vi "CIPT_softwarecontrol 24 7 23.vi"() -> ()   [LabVIEW 2022 SP3]
uses:
  CIPT modes.ctl
  <vilib>/Analysis/baseanly.llb/Mean (DBL).vi
  <vilib>/Utility/file.llb/Read Delimited Spreadsheet (DBL).vi
  <vilib>/Utility/file.llb/Read Delimited Spreadsheet (I64).vi
  <vilib>/gmath/NumericalOptimization/Nonlinear Curve Fit LM.vi
  <vilib>/Utility/file.llb/Write Delimited Spreadsheet (string).vi
  C:/CIPT/Labview Project/Camera Driver/Labview Driver/OtherDrivers/LabVIEW/ueye.NET/uEyeDotNet.dll
  CIPT/Labview Project/Camera Driver/Labview Driver/OtherDrivers/LabVIEW/ueye.NET/uEyeDotNet.dll
  <vilib>/Utility/file.llb/Write Delimited Spreadsheet (DBL).vi
  <vilib>/Utility/file.llb/Write Delimited Spreadsheet (I64).vi
  <vilib>/gmath/NI_Gmath.lvlib
  <instrlib>/Keithley DMM6500 DAQ6500 Series/Keithley DMM6500 DAQ6500 Series.lvlib
  <instrlib>/Keithley 24XX/Keithley 24XX.lvlib
  <instrlib>/Keithley 2182/Keithley 2182.lvlib
  <vilib>/Analysis/NI_AALBase.lvlib
panel:
  out "Comms Errors":errorcluster[](array[cluster])
  in  "Save Filr":bool
  out "error file out":errorcluster
  in  "output file path":path=path "C:/CIPT/Labview Project/csv files/test output.csv"
  in  "stop":bool
  in  "Tab Control":T1(tab)
  in  "Camera ID 3":enum16{"2", "1"}(ring)
  in  "Camera ID 1":enum16{"2", "1"}(ring)
  in  "down a2":bool
  in  "up a2":bool
  in  "down a1":bool
  in  "up a1":bool
  in  "down a3":bool
  in  "up a3":bool
  in  "down all":bool
  in  "up all":bool
  in  "steps /\n continuous \ntoggle":bool
  out "Image first camera":picture
  out "Serial Number 1":string
  in  "Init Camera":bool
  in  "Exit Camera":bool
  in  "Init Camera 2":bool
  in  "Exit Camera 2":bool
  out "Serial Number 2":string
  out "Image second camera":picture
  out "Error Camera 1":errorcluster caption="error"
  out "Error Camera 2":errorcluster caption="error"
  in  "COM 1":refnum<visa-resource-name>
  out "error":errorcluster
  in  "Probe Landing File":path=path "C:/CIPT/Labview Project/csv files/Probe Landing cipt.csv"
  in  "Landing Test on/off?":bool
  in  "load file":bool
  in  "Step size":i32=10
  out "Resistance":dbl[][](array[numeric])
  out "Measurment":sgl[](array[numeric])
  out "Loaded":bool
  out "Loaded":bool
  out "Error Probe Configuration File":errorcluster
  in  "Probe Configuration File":path=path "C:/CIPT/Labview Project/csv files/test probe config.csv"
  in  "Probe Settings File":path=path "C:/CIPT/Labview Project/csv files/deafult_probe_setrings.CSV"
  out "Error Probe Settings File":errorcluster
  out "Probe Spacings":dbl[][](array[numeric])
  in  "Load":bool
  in  "Multiplexer":refnum<visa-resource-name>
  out "all rows":i64[][](array[numeric])
  out "Results Description":string[](array[string])
  out "Results":dbl[][](array[numeric])
  out "Probe Set 2":i32
  in  "Compliance voltage (V)":dbl=42.0
  in  "Measure Instrument":refnum<visa-resource-name>
  in  "Radio Buttons":T2 caption="Select Instrumentation"
  in  "Source Instrument":refnum<visa-resource-name>
  in  "Run":bool
  in  "Current (µA)":dbl=10.0
  out "Measurement Log":string
  out "Probe Set":i32
  in  "Measurement Repeats":i32=10
  in  "Top Film R est.":dbl=0.25
  in  "Bottm Film R est.":dbl=0.25
  in  "RA est.":dbl=0.25
  out "Top Film R":dbl
  out "Bottom Film R":dbl
  out "RA":dbl
  out "error out (fitting model)":errorcluster
  in  "Fit Data":bool
  out "Measurements Map Out":map{string, dbl[]}(c390)
  # "Probe Landing cipt_probe check: checks probes individually \nProbe Landing cipt: checks for any connection"
  # "All"
  # "End"
  # "home"
  # "Delete"
  # "Insert"
  # "Page Down"
  # "Page up"
  # "F2"
  # "F1"
  # "Steps"
  # "Continuous"
  # "Probe Settings"
  # "Probe Configuration"
  # "I+"
  # "V+"
  # "V-"
  # "I-"
  # "Max Resolution of 2400 is 300 µV in 200 mV range"
  # "/"
  # "Sheet Resistance (RA)"
  # "Estimated Values"
  # "Fitted Values"
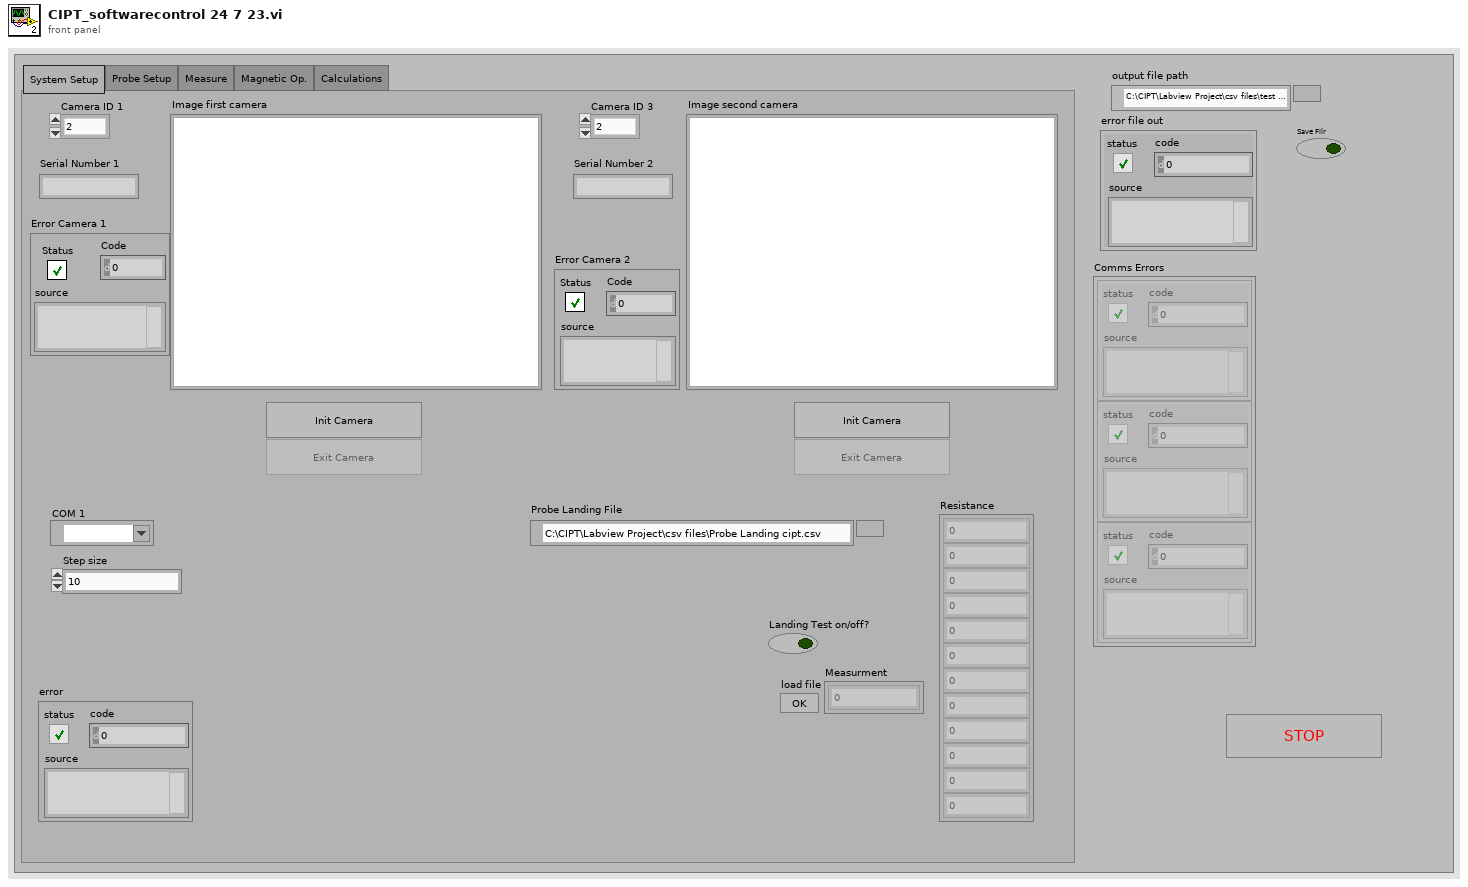
[diagram p1: front panel]
types:
  T1 = enum32{"System Setup", "Probe Setup", "Measure", "Magnetic Op.", "Calculations"}
  T2 = typedef "CIPT modes.ctl" = enum32{"DAQ6510", "2400 Only", "2400 and  2182", "SR830", "SR830 and 6221"}
  T3 = enum32{"System Setup", "Probe Setup", "Measure", "Magnetic Operations", "Calculations + Analyis"}
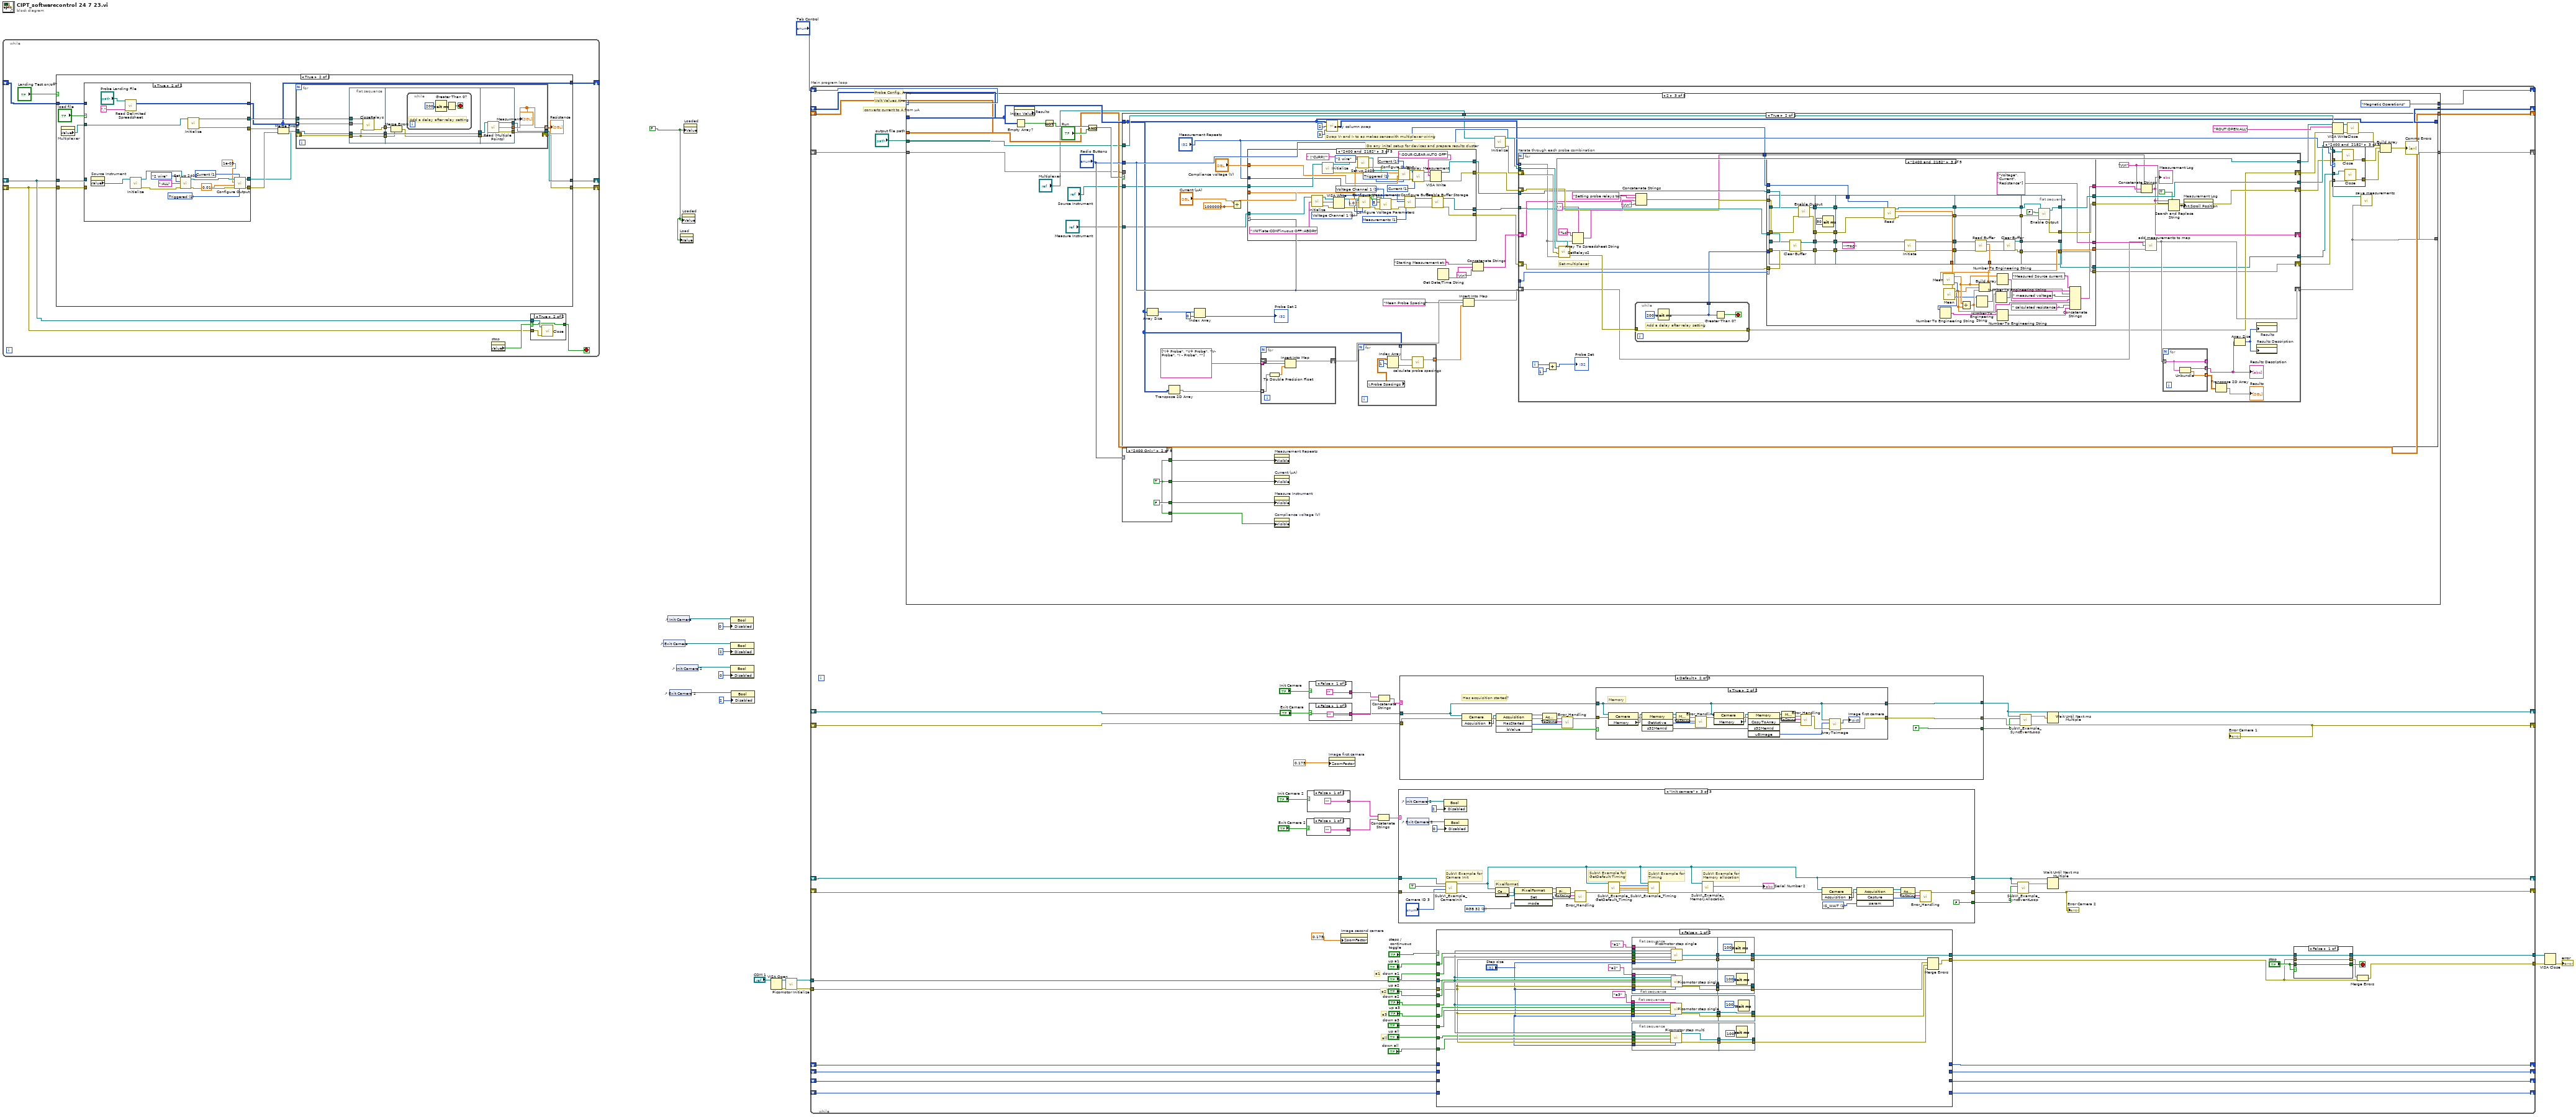
[diagram p0: block diagram]
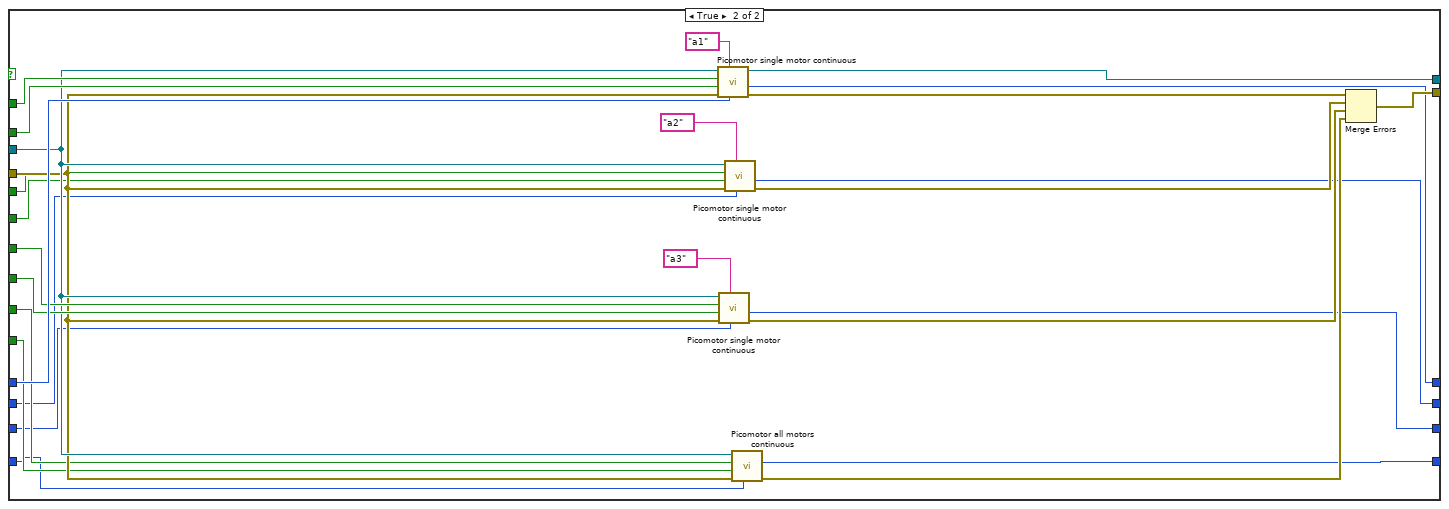
[diagram p5: hidden frame]
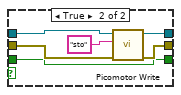
[diagram p6: hidden frame]
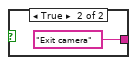
[diagram p7: hidden frame]
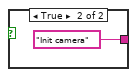
[diagram p8: hidden frame]
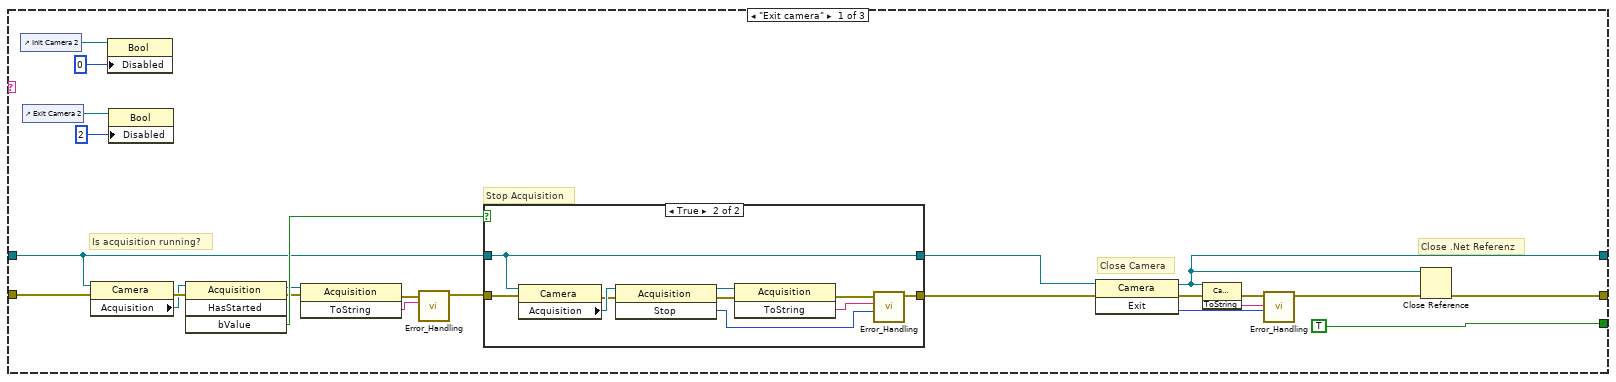
[diagram p9: hidden frame]
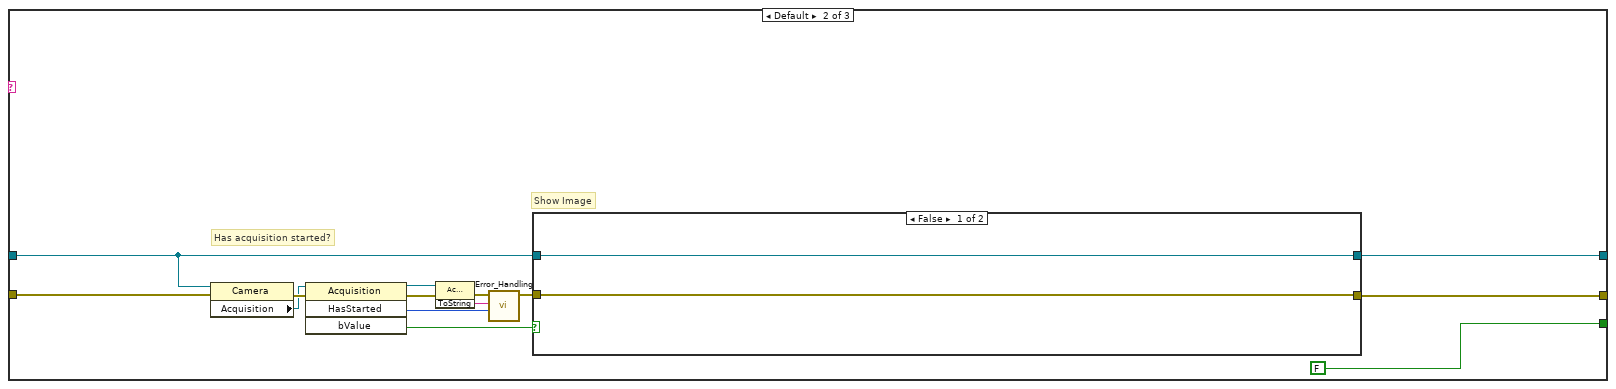
[diagram p11: hidden frame]
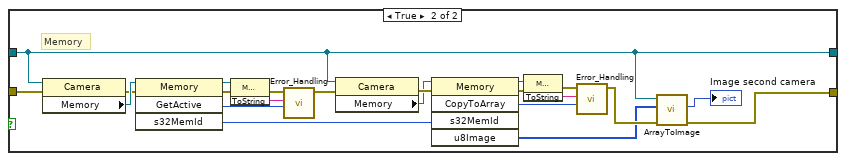
[diagram p12: hidden frame]
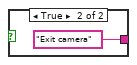
[diagram p13: hidden frame]
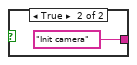
[diagram p14: hidden frame]
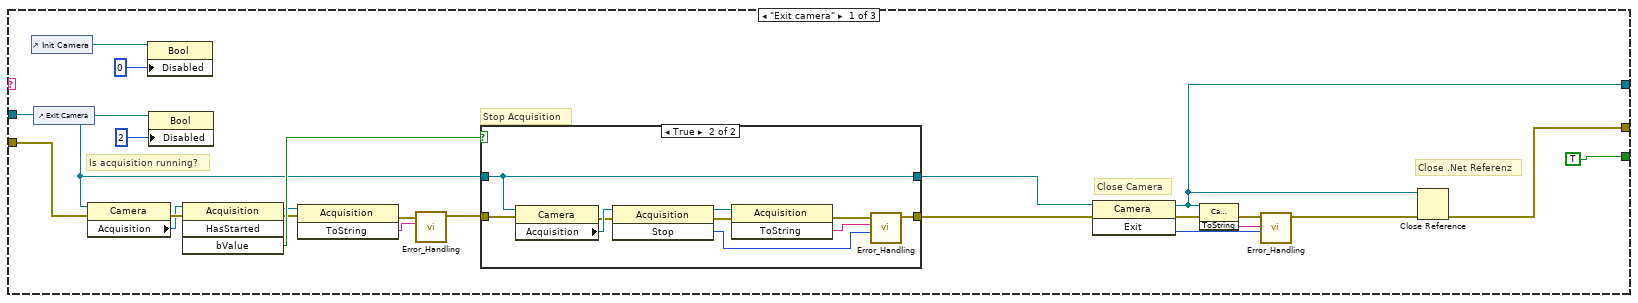
[diagram p15: hidden frame]
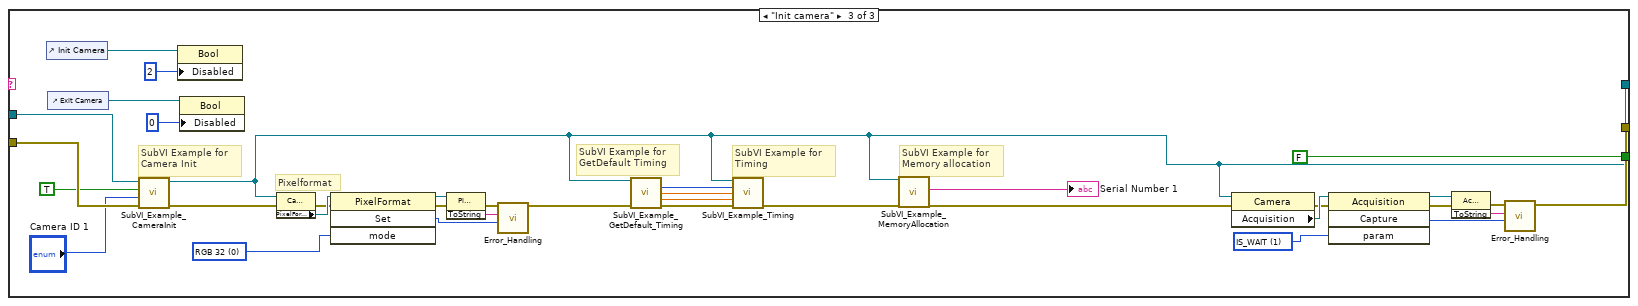
[diagram p18: hidden frame]
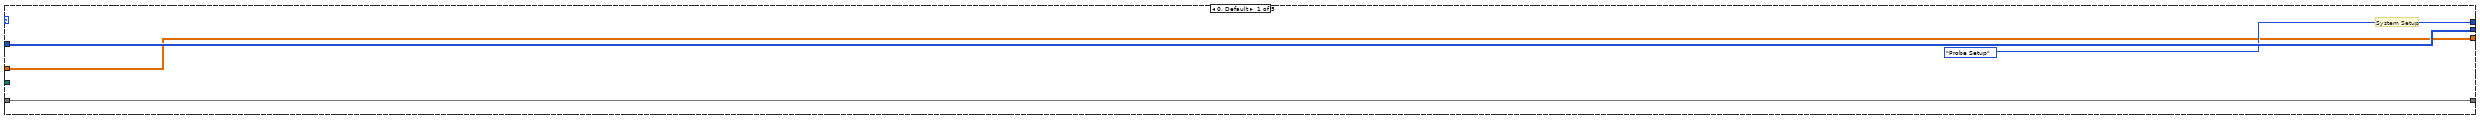
[diagram p19: hidden frame]
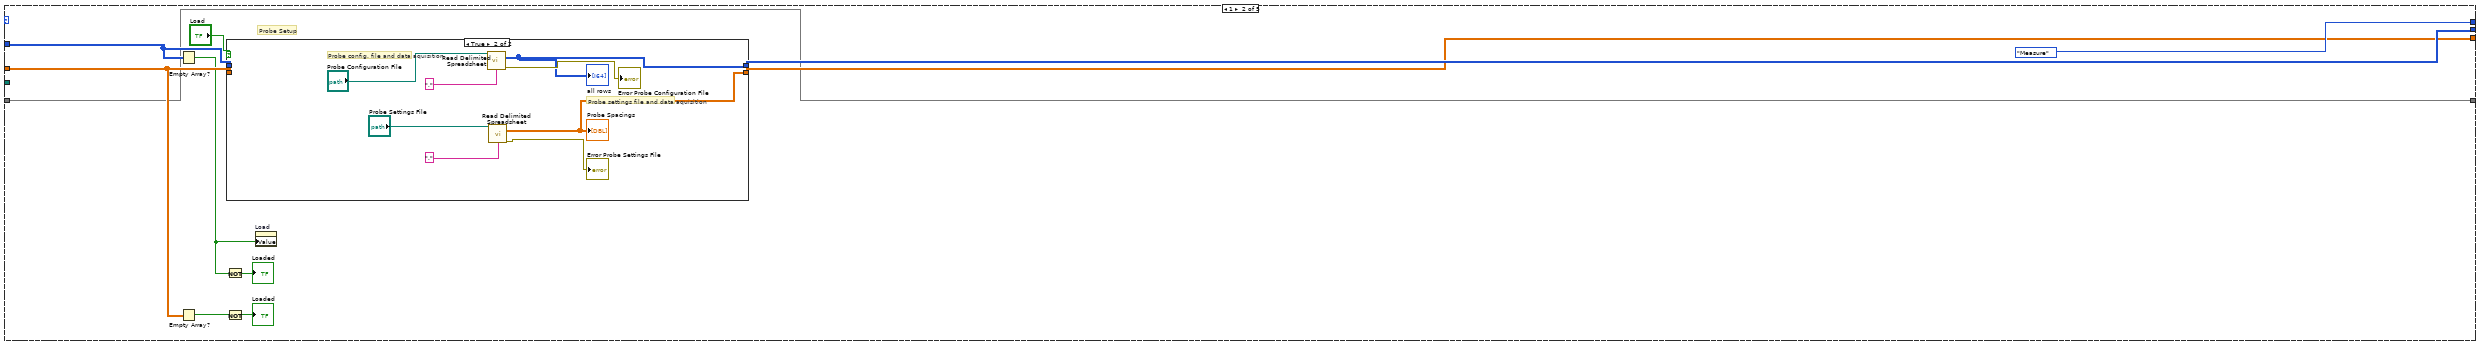
[diagram p20: hidden frame]
diagram:
  w9 = FALSE
  n1 = while {
    shift-right: [w26] -> _
    shift-left: _ -> [w23]
    shift-right: [w25] -> _
    shift-left: _ -> [w22]
    shift-right: [w20] -> _
    shift-left: _ -> [w19]
    stop <- w21 stop-if-true
    n2 = case shown="True" "Landing Test on/off?" {
      tunnel: w23 -> [w34 w43]
      tunnel: w22 -> [w33 w42]
      tunnel: [w34 w41] -> w26
      tunnel: [w33 w40] -> w25
      tunnel: w19 -> [w32 w36]
      tunnel: [w32 w35] -> w20
      frame False {
      }
      frame True {
        n3 = property on="Multiplexer" class="VISAName"() -> ("Value"=w39:refnum<visa-resource-name>)  [unwired: 2 in, 2 out]
        n4 = case shown="True" "load file" {
          tunnel: [_ w84] -> w48
          tunnel: [w80 w87] -> w45
          tunnel: [w81 w86] -> w44
          tunnel: w43 -> [w81 _]
          tunnel: w42 -> [w80 _]
          tunnel: [w79 w85] -> w38
          tunnel: w39 -> [w79 w83]
          tunnel: [w78 w82] -> w35
          tunnel: w36 -> [w78 _]
          frame False {
          }
          frame True {
            w93 = u16 1 items=["Immediate", "Triggered"] ("Output Type  (0: Immediate)")
            w92 = u16 1 items=["Voltage", "Current"] ("Source Mode  (0: Voltage)")
            n5 = property on="Source Instrument" class="VISAName"() -> ("Value"=w98:refnum<visa-resource-name>)  [unwired: 2 in, 2 out]
            n6 = call-poly <vilib>:"Read Delimited Spreadsheet.vi"("file path (dialog if empty)"="Probe Landing File", "delimiter (\\t)"="," ("delimiter (\\t)")) -> ("all rows"=w82:i64[][])  [unwired: 8 in, 5 out]
            n7 = call <instrlib>:"Initialize.vi"("VISA resource name"=w98) -> ("error out"=w95:errorcluster, "VISA resource name out"=w94:refnum<visa-resource-name>)  [unwired: 9 in]
            n8 = call "Set up 2400.vi"("VISA resource name"=w94, "Sense mode"=enum16{"2 wire", "4 wire"}."2 wire", "Measurement Function"=":ALL", "error in (no error)"=w95) -> ("VISA resource name out"=w96:refnum<visa-resource-name>, "error out"=w97:errorcluster)  [unwired: 10 in]
            n9 = call <instrlib>:"Initialize.vi"("VISA resource name"=w83) -> ("error out"=w84:errorcluster, "VISA resource name out"=w85:refnum<visa-resource-name>)  [unwired: 9 in]
            n10 = call <instrlib>:"Configure Output.vi"("Output Type  (0: Immediate)"=w93, "Source Mode  (0: Voltage)"=w92, "error in (no error)"=w97, "Compliance  Level (0.1)"=0.01, "Output Level (0)"=1e-05, "VISA resource name"=w96) -> ("error out"=w87:errorcluster, "VISA resource name out"=w86:refnum<visa-resource-name>)  [unwired: 4 in]
          }
        }
        n11 = Merge Errors(w48, w45) -> (w47:errorcluster)
        n12 = for {
          tunnel: [w54] -> w37 mode=indexing
          tunnel: w38 -> [w50]
          shift-right: [w51] -> w40
          shift-left: w47 -> [w55]
          tunnel: w35 -> [w49] mode=indexing
          tunnel: w44 -> [w53]
          tunnel: [w52] -> w41
          n13 = flat-sequence {
            tunnel: w53 -> [w65]
            tunnel: w55 -> [w61]
            tunnel: [w61] -> w60
            tunnel: [w65] -> w59
            tunnel: w50 -> [w64]
            tunnel: [w63] -> w58
            tunnel: w49 -> [w62]
            tunnel: [w67] -> w57
            tunnel: [w69] -> w56
            tunnel: w60 -> [w68]
            tunnel: w59 -> [w69]
            tunnel: w58 -> [w66]
            tunnel: [w75] -> w54
            tunnel: [w74] -> w52
            tunnel: [w73] -> w51
            tunnel: w57 -> [w77]
            tunnel: w56 -> [w76]
            frame #0 {
              n14 = call "CloseRelays.vi"("error in (no error)"=w61, "Array"=w62, "VISA Refnum in"=w64) -> ("error out"=w63:errorcluster)  [unwired: 6 in, 2 out]
            }
            frame #1 {
              n15 = Merge Errors(w66, w68) -> (w67:errorcluster)
              n16 = while {
                stop <- w71 stop-if-true
                # "Add a delay after relay setting"
                n17 = Wait (ms)(milliseconds to wait=u32 200) -> (millisecond timer value=w70:u32)
                n18 = Greater Than 0?(x=w70) -> (x > 0?=w71:bool)
              }
            }
            frame #2 {
              n19 = call <instrlib>:"Read (Multiple Points).vi"("VISA resource name"=w76, "error in (no error)"=w77) -> ("VISA resource name out"=w74:refnum<visa-resource-name>, "Resistance"=w75:sgl[], "error out"=w73:errorcluster)  [unwired: 7 in, 4 out]
            }
          }
          "Measurment" <- w54
        }
        "Resistance" <- w37
      }
    }
    n20 = property on="stop" class="Bool (strict)"() -> ("Value"=w24:bool)  [unwired: 2 in, 2 out]
    n21 = case shown="True" w24 {
      selector: w24 -> [w28 w29]
      tunnel: w23 -> [_ w31]
      tunnel: w22 -> [_ w30]
      tunnel: [w28 w29] -> w21
      frame False {
      }
      frame True {
        n22 = call <instrlib>:"Close.vi"("error in (no error)"=w30, "VISA resource name"=w31) -> ()  [unwired: 9 in, 1 out]
      }
    }
  }
  n23 = control-ref of="Exit Camera"() -> (w12:refnum<vi>)
  n24 = control-ref of="Init Camera"() -> (w13:refnum<vi>)
  n25 = control-ref of="Exit Camera 2"() -> (w17:refnum<vi>)
  n26 = control-ref of="Init Camera 2"() -> (w16:refnum<vi>)
  n27 = property on="Load" class="Bool (strict)"("Value"=w9) -> ()  [unwired: 2 in, 2 out]
  n28 = property on="Loaded" class="Bool (strict)"("Value"=w9) -> ()  [unwired: 2 in, 2 out]
  n29 = property on="Loaded" class="Bool (strict)"("Value"=w9) -> ()  [unwired: 2 in, 2 out]
  n30 = property class="Bool"(reference=w13, "Disabled"=u8 0 ("Deaktiviert")) -> ()  [unwired: 1 in, 2 out]
  n31 = property class="Bool"(reference=w12, "Disabled"=u8 2 ("Deaktiviert")) -> ()  [unwired: 1 in, 2 out]
  n32 = property class="Bool"(reference=w16, "Disabled"=u8 0 ("Deaktiviert")) -> ()  [unwired: 1 in, 2 out]
  n33 = property class="Bool"(reference=w17, "Disabled"=u8 2 ("Deaktiviert")) -> ()  [unwired: 1 in, 2 out]
  n34 = VISA Open(VISA resource name="COM 1") -> (VISA resource name=w7:refnum<visa-resource-name>, error out=w6:errorcluster)  [unwired: 4 in]
  n35 = call "Picomotor Initialize.vi"("error in (no error)"=w6, "VISA Refnum in"=w7) -> ("error out"=w4:errorcluster, "VISA Refnum out"=w5:refnum<visa-resource-name>)  [unwired: 8 in]
  n36 = while "Main program loop" {
    shift-right: [w159] -> _
    shift-left: _ -> [w160]
    shift-right: [w158] -> _
    shift-left: "Tab Control" -> [w161]
    shift-right: [w157] -> _
    shift-left: _ -> [w156]
    shift-right: [w154] -> _
    shift-left: _ -> [w153]
    shift-right: [w142] -> _
    shift-left: _ -> [w140]
    shift-right: [w143] -> _
    shift-left: _ -> [w141]
    shift-right: [w130] -> _
    shift-left: _ -> [w128]
    shift-right: [w129] -> _
    shift-left: _ -> [w127]
    tunnel: w5 -> [w114]
    tunnel: w4 -> [w113]
    tunnel: [w126] -> w2
    shift-right: [w111] -> _
    shift-left: _ -> [w107]
    shift-right: [w110] -> _
    shift-left: _ -> [w106]
    shift-right: [w109] -> _
    shift-left: _ -> [w105]
    shift-right: [w108] -> _
    shift-left: _ -> [w104]
    tunnel: [w101] -> w1
    stop <- w125 stop-if-true
    # "a2"
    # "a3"
    # "all"
    # "a1"
    # "converts current to A from µA"
    # "Volt Values Array"
    # "Probe Config. Array"
    n37 = case shown="2" w161 {
      tunnel: w160 -> [w500 w507 w536 w840 w847]
      tunnel: [w500 w511 w535 w840 w847] -> w159
      tunnel: [T3."Probe Setup" ("Tab Control") T3."Measure" ("Tab Control") T3."Magnetic Operations" ("Tab Control") T3."Calculations + Analyis" ("Tab Control") T3."System Setup" ("Tab Control")] -> w158
      tunnel: [w498 w506 w530 w839 w846] -> w157
      tunnel: w156 -> [w498 w505 w530 w839 w846]
      tunnel: "output file path" -> [_ _ w527 _ w845]
      tunnel: [w497 w502 w526 w838 w844] -> w154
      tunnel: w153 -> [w497 w502 w525 w838 w844]
      frame 0, Default {
        # "System Setup"
      }
      frame 1 {
        # "Probe Setup"
        n38 = Empty Array?(array=w507) -> (empty?=w501:bool)
        n39 = Empty Array?(array=w505) -> (empty?=w504:bool)
        n40 = Not(x=w501) -> (.not. x?=→"Loaded":bool)
        n41 = Not(x=w504) -> (.not. x?=→"Loaded":bool)
        n42 = case shown="True" "Load" {
          tunnel: [w513 w514] -> w511
          tunnel: w507 -> [w513 _]
          tunnel: [w512 w515] -> w506
          tunnel: w505 -> [w512 _]
          frame False {
          }
          frame True {
            # "Probe config. file and data aquisition"
            # "Probe settings file and data aquisition"
            n43 = call-poly <vilib>:"Read Delimited Spreadsheet.vi"("file path (dialog if empty)"="Probe Configuration File", "delimiter (\\t)"="," ("delimiter (\\t)")) -> ("all rows"=w514:i64[][], "error out"=→"Error Probe Configuration File":errorcluster)  [unwired: 8 in, 4 out]
            "all rows" <- w514
            n44 = call-poly <vilib>:"Read Delimited Spreadsheet.vi"("file path (dialog if empty)"="Probe Settings File", "delimiter (\\t)"="," ("delimiter (\\t)")) -> ("all rows"=w515:dbl[][], "error out"=→"Error Probe Settings File":errorcluster)  [unwired: 8 in, 4 out]
            "Probe Spacings" <- w515
          }
        }
        n45 = property on="Load" class="Bool (strict)"("Value"=w501) -> ()  [unwired: 2 in, 2 out]
      }
      frame 2 {
        n46 = property on="Results" class="Arr (strict)" props=["Index Values"]() -> ()  [unwired: 2 in, 3 out]
        n47 = Empty Array?(array=w536) -> (empty?=w538:bool)
        n48 = Not(x=w538) -> (.not. x?=w537:bool)
        n49 = Compound Arithmetic op=AND(w537, "Run") -> (w540:bool)
        n50 = case shown="True" w540 {
          tunnel: w536 -> [w551 w567]
          tunnel: [w551 w567] -> w535
          tunnel: "Radio Buttons" -> [_ w595]
          tunnel: w527 -> [_ w582]
          tunnel: [w550 w562] -> w526
          tunnel: w525 -> [w550 _]
          tunnel: "Measure Instrument" -> [_ w554]
          tunnel: "Source Instrument" -> [_ w553]
          tunnel: "Multiplexer" -> [_ w552]
          frame False {
          }
          frame True {
            # "Swap V- and I- to as makes sensewith multiplexer wiring"
            # "Do any inital setup for devices and prepare results cluster"
            n51 = Array Size(array=w567) -> (size(s)=w588:i32[])
            n52 = Transpose 2D Array(2D array=w567) -> (transposed array=w566:i64[][])
            n53 = Index Array "Index Array"(array=w588, index=0) -> (element=→"Probe Set 2":i32)
            n54 = Divide(x="Current (µA)", y=1000000.0) -> (x/y=w573:dbl)
            n55 = case shown="\"2400 and  2182\"" w595 {
              tunnel: w553 -> [_ w633 w660 _ _]
              tunnel: [_ w621 w644 _ _] -> w596
              tunnel: w554 -> [_ _ w659 _ _]
              tunnel: [_ w621 w652 _ _] -> w556
              tunnel: [_ w627 w651 _ _] -> w590
              tunnel: w573 -> [_ w624 w669 _ _]
              tunnel: "Compliance voltage (V)" -> [_ w622 w670 _ _]
              tunnel: [_ _ w643 _ _] -> w565
              tunnel: "Measurement Repeats" -> [_ _ w647 _ _]
              frame "DAQ6510", Default {
              }
              frame "2400 Only" {
                w625 = u16 1 items=["Immediate", "Triggered"] ("Output Type  (0: Immediate)")
                w626 = u16 1 items=["Voltage", "Current"] ("Source Mode  (0: Voltage)")
                n56 = call <instrlib>:"Initialize.vi"("VISA resource name"=w633) -> ("error out"=w631:errorcluster, "VISA resource name out"=w632:refnum<visa-resource-name>)  [unwired: 9 in]
                n57 = call "Set up 2400.vi"("VISA resource name"=w632, "Sense mode"=enum16{"2 wire", "4 wire"}."4 wire", "Measurement Function"=":ALL", "error in (no error)"=w631) -> ("VISA resource name out"=w629:refnum<visa-resource-name>, "error out"=w628:errorcluster)  [unwired: 10 in]
                n58 = call <instrlib>:"Configure Output.vi"("Output Type  (0: Immediate)"=w625, "Source Mode  (0: Voltage)"=w626, "error in (no error)"=w628, "Compliance  Level (0.1)"=w622, "Output Level (0)"=w624, "VISA resource name"=w629) -> ("error out"=w627:errorcluster, "VISA resource name out"=w621:refnum<visa-resource-name>)  [unwired: 4 in]
              }
              frame "2400 and  2182" {
                w635 = 1 items=["Voltage Channel 1"=1, "Voltage Channel 2"=2] ("Measurement (1: Voltage Channel 1)")
                w649 = 1 items=["None", "Measurements", "Math Calculation"] ("Buffer Source (0: None)")
                w656 = u16 1 items=["Voltage", "Current", "Resistance"] ("Displayed Measurement (0: Voltage)")
                w665 = u16 1 items=["Voltage", "Current"] ("Source Mode  (0: Voltage)")
                w668 = u16 1 items=["Immediate", "Triggered"] ("Output Type  (0: Immediate)")
                w673 = 0 items=["Voltage Channel 1", "Voltage Channel 2", "Temperature Channel 1", "Temperature Channel 2"] ("Measurement (0: Voltage Channel 1)")
                n59 = call <instrlib>:"Initialize.vi"("VISA resource name"=w659) -> ("error out"=w642:errorcluster, "VISA resource name out"=w640:refnum<visa-resource-name>)  [unwired: 9 in]
                n60 = call <instrlib>:"Initialize.vi"("VISA resource name"=w660) -> ("error out"=w662:errorcluster, "VISA resource name out"=w667:refnum<visa-resource-name>)  [unwired: 9 in]
                n61 = VISA Write(VISA resource name=w640, write buffer=":INITiate:CONTinuous OFF;:ABORt", error in (no error)=w642) -> (VISA resource name out=w639:refnum<visa-resource-name>, error out=w641:errorcluster)  [unwired: 1 out]
                n62 = call "Set up 2400.vi"("VISA resource name"=w667, "Sense mode"=enum16{"2 wire", "4 wire"}."2 wire", "Measurement Function"=" \"CURR\"", "error in (no error)"=w662) -> ("VISA resource name out"=w666:refnum<visa-resource-name>, "error out"=w661:errorcluster)  [unwired: 10 in]
                n63 = call <instrlib>:"Configure Measurements.vi"("VISA resource name"=w639, "Measurement (0: Voltage Channel 1)"=w673, "Integration Rate (5)"=1.0, "error in (no error)"=w641, "Sample Count (1)"=w647) -> ("VISA resource name out"=w671:refnum<visa-resource-name>, "error out"=w672:errorcluster)  [unwired: 9 in]
                n64 = call <instrlib>:"Configure Voltage Parameters.vi"("VISA resource name"=w671, "Measurement (1: Voltage Channel 1)"=w635, "Voltage Resolution (8)"=8, "Autorange (T: Enable)"=TRUE, "error in (no error)"=w672) -> ("VISA resource name out"=w648:refnum<visa-resource-name>, "error out"=w650:errorcluster)  [unwired: 9 in]
                n65 = call <instrlib>:"Configure Output.vi"("Output Type  (0: Immediate)"=w668, "Source Mode  (0: Voltage)"=w665, "error in (no error)"=w661, "Compliance  Level (0.1)"=w670, "Output Level (0)"=w669, "VISA resource name"=w666) -> ("error out"=w657:errorcluster, "VISA resource name out"=w658:refnum<visa-resource-name>)  [unwired: 4 in]
                n66 = call <instrlib>:"Configure Buffer.vi"("error in (no error)"=w650, "Buffer Source (0: None)"=w649, "Buffer Size (2)"=w647, "VISA resource name"=w648) -> ("error out"=w646:errorcluster, "VISA resource name out"=w645:refnum<visa-resource-name>)  [unwired: 6 in]
                n67 = call <instrlib>:"Display Measurement.vi"("error in (no error)"=w657, "Displayed Measurement (0: Voltage)"=w656, "VISA resource name"=w658) -> ("error out"=w655:errorcluster, "VISA resource name out"=w654:refnum<visa-resource-name>)  [unwired: 7 in]
                n68 = VISA Write(VISA resource name=w654, write buffer=":SOUR:CLEAR:AUTO OFF", error in (no error)=w655) -> (VISA resource name out=w652:refnum<visa-resource-name>, error out=w651:errorcluster)  [unwired: 1 out]
                n69 = call <instrlib>:"Enable Buffer Storage.vi"("error in (no error)"=w646, "VISA resource name"=w645) -> ("error out"=w643:errorcluster, "VISA resource name out"=w644:refnum<visa-resource-name>)  [unwired: 8 in]
              }
              frame "SR830" {
              }
              frame "SR830 and 6221" {
              }
            }
            n70 = for {
              tunnel: w566 -> [w607] mode=indexing
              tunnel: string[] ["I+ Probe", "V+ Probe", "V- Probe", "I - Probe", ""] -> [w608] mode=indexing
              shift-right: [w605] -> w571
              shift-left: _ -> [w604]
              n71 = To Double Precision Float(number=w607) -> (double precision float=w606:dbl[])
              n72 = Insert Into Map(map in=w604, key=w608, value=w606) -> (map out=w605:map{string, dbl[]})  [unwired: 2 out]
            }
            n73 = call "array column swap.vi"("Collumn 2 index"=3, "Collumn 1 index"=2, "Input array"=w567) -> ("output array"=w585:i32[][])
            n74 = for {
              tunnel: w567 -> [w600] mode=indexing
              tunnel: [w599] -> w570 mode=indexing
              n75 = local read "Probe Spacings"() -> (w603:dbl[][])
              n76 = Index Array(array=w603, index (row)=1) -> (element=w601:dbl[])  [unwired: 1 in]
              n77 = call "calculate probe spacings.vi"("Probe Spacings"=w601, "Probe list"=w600) -> ("Mean Spacing"=w599:dbl)  [unwired: 1 out]
            }
            n78 = Get Date/Time String() -> (time string=w592:string)  [unwired: 3 in, 1 out]
            n79 = Insert Into Map(map in=w571, key="Mean Probe Spacing", value=w570) -> (map out=w568:map{string, dbl[]})  [unwired: 2 out]
            n80 = Concatenate Strings("Starting Measurement at: ", w592, "\r\n") -> (w580:string)
            n81 = call <instrlib>:"Initialize.vi"("VISA resource name"=w552) -> ("error out"=w597:errorcluster, "VISA resource name out"=w598:refnum<visa-resource-name>)  [unwired: 9 in]
            n82 = for "Iterate through each probe combination" {
              tunnel: w598 -> [w713]
              tunnel: [w712] -> w578
              tunnel: w585 -> [w706] mode=indexing
              tunnel: w595 -> [w711]
              tunnel: w596 -> [w709]
              shift-right: [w695] -> _
              shift-left: w580 -> [w696]
              shift-right: [w707] -> w593
              shift-left: w590 -> [w700]
              shift-right: [w686] -> w562
              shift-left: w568 -> [w688]
              shift-right: [w679] -> w563
              shift-left: w565 -> [w680]
              tunnel: w556 -> [w699]
              tunnel: [w708] -> w594
              shift-right: [w682] -> w558
              shift-left: w597 -> [w710]
              tunnel: [w678] -> w564
              tunnel: "Measurement Repeats" -> [w677]
              i -> [w676]
              w693 = "\r\n"
              # "Set multiplexer"
              n83 = Add(x=w676, y=1) -> (x+y=→"Probe Set":i32)
              n84 = call "SetRelays2.vi"("all rows"=w706, "error in (no error)"=w710, "VISA Refnum in"=w713) -> ("error out"=w701:errorcluster, "VISA resource name out"=w712:refnum<visa-resource-name>)  [unwired: 1 in]
              n85 = Array To Spreadsheet String(delimiter (Tab)=",", array=w706, 3:"%d" ("format string")) -> (spreadsheet string=w702:string)
              n86 = while {
                tunnel: [w720] -> w682
                tunnel: w701 -> [w720]
                tunnel: [w717] -> w681
                stop <- w718 stop-if-true
                # "Add a delay after relay setting"
                n87 = Wait (ms)(milliseconds to wait=u32 200) -> (millisecond timer value=w717:u32)
                n88 = Greater Than 0?(x=w717) -> (x > 0?=w718:bool)
              }
              n89 = Concatenate Strings(w696, "Setting probe relays to:", w702, "\r\n") -> (w691:string)
              n90 = case shown="\"2400 and  2182\"" w711 {
                tunnel: w709 -> [w722 w726 w775 w830 w834]
                tunnel: w699 -> [w721 w747 w790 w831 w835]
                tunnel: w700 -> [w723 w746 w789 w832 w836]
                tunnel: [w721 w744 w788 w831 w835] -> w708
                tunnel: [w723 w743 w785 w832 w836] -> w707
                tunnel: [_ w736 w780 _ _] -> w697
                tunnel: w677 -> [_ w735 w787 _ _]
                tunnel: [_ w729 w784 _ _] -> w689
                tunnel: [_ string[] ["Voltage", "Current", "Resistance"] string[] ["Voltage", "Current", "Resistance"] _ _] -> w690
                tunnel: w681 -> [_ _ _ _ _]
                tunnel: w680 -> [w724 w727 w774 w833 w837]
                tunnel: [w724 w727 w776 w833 w837] -> w679
                tunnel: [w722 w726 w777 w830 w834] -> w678
                frame "DAQ6510", Default {
                }
                frame "2400 Only" {
                  w745 = u16 0 items=["Fixed", "Sweep", "List"] ("Output Mode (0: Fixed)")
                  n91 = call <instrlib>:"Read (Multiple Points).vi"("VISA resource name"=w747, "Sample Count (1)"=w735, "error in (no error)"=w746, "Output Mode (0: Fixed)"=w745) -> ("Voltage"=w725:sgl[], "VISA resource name out"=w744:refnum<visa-resource-name>, "Current"=w734:sgl[], "Resistance"=w733:sgl[], "error out"=w743:errorcluster)  [unwired: 5 in, 2 out]
                  n92 = call-poly <vilib>:"Mean.vi"("X"=w725) -> ("mean"=w732:dbl)  [unwired: 1 out]
                  n93 = call-poly <vilib>:"Mean.vi"("X"=w734) -> ("mean"=w731:dbl)  [unwired: 1 out]
                  n94 = call-poly <vilib>:"Mean.vi"("X"=w733) -> ("mean"=w730:dbl)  [unwired: 1 out]
                  n95 = Build Array(w732, w731, w730) -> (w729:dbl[])
                  n96 = Number To Engineering String(4:w732) -> (0:w737:string)  [unwired: 3 in]
                  n97 = Number To Engineering String(4:w731) -> (0:w741:string)  [unwired: 3 in]
                  n98 = Number To Engineering String(4:w730) -> (0:w738:string)  [unwired: 3 in]
                  n99 = Concatenate Strings("Measured I = ", w741, " V = " ("string"), w737, "R = " ("string"), w738) -> (w736:string)
                }
                frame "2400 and  2182" {
                  n100 = flat-sequence {
                    tunnel: w790 -> [w798]
                    tunnel: w789 -> [w797]
                    tunnel: [w796] -> w755
                    tunnel: [w795] -> w753
                    tunnel: w775 -> [w794]
                    tunnel: w774 -> [w791]
                    tunnel: [w793] -> w751
                    tunnel: [w792] -> w749
                    tunnel: w755 -> [w803]
                    tunnel: [w803] -> w754
                    tunnel: w753 -> [w802]
                    tunnel: [w802] -> w752
                    tunnel: w751 -> [w801]
                    tunnel: [w801] -> w750
                    tunnel: w749 -> [w800]
                    tunnel: [w800] -> w748
                    tunnel: w754 -> [w813]
                    tunnel: w752 -> [w812]
                    tunnel: w787 -> [w811]
                    tunnel: [w810] -> w779
                    tunnel: [w809] -> w778
                    tunnel: [w808] -> w767
                    tunnel: w750 -> [w807]
                    tunnel: w748 -> [w806]
                    tunnel: [w805] -> w773
                    tunnel: [w804] -> w772
                    tunnel: w779 -> [w815]
                    tunnel: w778 -> [w814]
                    tunnel: [w822] -> w756
                    tunnel: w773 -> [w817]
                    tunnel: w772 -> [w816]
                    tunnel: [w820] -> w771
                    tunnel: [w818] -> w770
                    tunnel: [w815] -> w769
                    tunnel: [w814] -> w768
                    tunnel: [w828] -> w776
                    tunnel: [w829] -> w777
                    tunnel: [w825] -> w785
                    tunnel: [w824] -> w788
                    tunnel: w771 -> [w829]
                    tunnel: w770 -> [w828]
                    tunnel: w769 -> [w827]
                    tunnel: w768 -> [w826]
                    frame #0 {
                      n101 = call <instrlib>:"Clear Buffer.vi"("error in (no error)"=w791, "VISA resource name"=w794) -> ("error out"=w792:errorcluster, "VISA resource name out"=w793:refnum<visa-resource-name>)  [unwired: 8 in]
                      n102 = call <instrlib>:"Enable Output.vi"("error in (no error)"=w797, "VISA resource name"=w798) -> ("error out"=w795:errorcluster, "VISA resource name out"=w796:refnum<visa-resource-name>)  [unwired: 8 in]
                    }
                    frame #1 {
                      n103 = Wait (ms)(milliseconds to wait=u32 50) -> ()  [unwired: 1 out]
                    }
                    frame #2 {
                      (unwired) "*TRG" ("write buffer")
                      n104 = call-poly <instrlib>:"Read.vi"("VISA resource name"=w813, "Sample Count (1)"=w811, "error in (no error)"=w812) -> ("VISA resource name out"=w809:refnum<visa-resource-name>, "Current"=w808:sgl[], "error out"=w810:errorcluster)  [unwired: 6 in, 4 out]
                      n105 = call <instrlib>:"Initiate.vi"("error in (no error)"=w806, "VISA resource name"=w807) -> ("error out"=w804:errorcluster, "VISA resource name out"=w805:refnum<visa-resource-name>)  [unwired: 8 in]
                    }
                    frame #3 {
                      n106 = call <instrlib>:"Read Buffer.vi"("error in (no error)"=w816, "VISA resource name"=w817) -> ("error out"=w819:errorcluster, "Buffer"=w822:dbl[], "VISA resource name out"=w821:refnum<visa-resource-name>)  [unwired: 6 in, 1 out]
                      n107 = call <instrlib>:"Clear Buffer.vi"("error in (no error)"=w819, "VISA resource name"=w821) -> ("error out"=w818:errorcluster, "VISA resource name out"=w820:refnum<visa-resource-name>)  [unwired: 8 in]
                    }
                    frame #4 {
                      n108 = call <instrlib>:"Enable Output.vi"("error in (no error)"=w827, "Enable Output (T: Enable)"=FALSE, "VISA resource name"=w826) -> ("error out"=w825:errorcluster, "VISA resource name out"=w824:refnum<visa-resource-name>)  [unwired: 7 in]
                    }
                  }
                  n109 = call-poly <vilib>:"Mean.vi"("X"=w756) -> ("mean"=w783:dbl, "error"=w760:i32)
                  n110 = Number To Engineering String(4:w760) -> (0:w759:string)  [unwired: 3 in]
                  n111 = call-poly <vilib>:"Mean.vi"("X"=w767) -> ("mean"=w782:dbl, "error"=w764:i32)
                  n112 = Divide(x=w783, y=w782) -> (x/y=w781:dbl)
                  n113 = Number To Engineering String(4:w764) -> (0:w763:string)  [unwired: 3 in]
                  n114 = Build Array(w783, w782, w781) -> (w784:dbl[])
                  n115 = Number To Engineering String(4:w782) -> (0:w765:string)  [unwired: 3 in]
                  n116 = Number To Engineering String(4:w781) -> (0:w757:string)  [unwired: 3 in]
                  n117 = Number To Engineering String(4:w783) -> (0:w761:string)  [unwired: 3 in]
                  n118 = Concatenate Strings("Measured Source current: " ("string"), w765, w763, " measured voltage: " ("string"), w761, w759, " calculated resistance: " ("string"), w757) -> (w780:string)
                }
                frame "SR830" {
                }
                frame "SR830 and 6221" {
                }
              }
              n119 = Concatenate Strings(w691, w697, w693) -> (w695:string)
              "Measurement Log" <- w695
              n120 = call "add measurements to map.vi"("Measurement Values"=w689, "Measurement Names"=w690, "Measurements Map in"=w688) -> ("Measurements Map Out"=w686:map{string, dbl[]})  [unwired: 2 in]
              n121 = for {
                tunnel: [w716] -> _ mode=indexing
                tunnel: w686 -> [w716] mode=indexing
                tunnel: [w715] -> w685 mode=indexing
                tunnel: [w714] -> w684 mode=indexing
                n122 = Unbundle(w716) -> (w715:string, "Array"=w714:dbl[])
              }
              "Results Description" <- w685
              n123 = Search and Replace String(replace all?=TRUE, input string=w695, search string=w693) -> (number of replacements=w692:i32)  [unwired: 5 in, 3 out]
              n124 = property on="Measurement Log" class="Str"("Text.Scroll Position"=w692) -> ()  [unwired: 2 in, 2 out]
              n125 = Transpose 2D Array(2D array=w684) -> (transposed array=→"Results":dbl[][])
              n126 = Array Size(array=w685) -> (size(s)=w687:i32)
              n127 = property on="Results" class="Arr (strict)"("Number of Columns"=w687) -> ()  [unwired: 2 in, 2 out]
              n128 = property on="Results Description" class="Arr (strict)"("Number of Columns"=w687) -> ()  [unwired: 2 in, 2 out]
            }
            n129 = VISA Write(VISA resource name=w578, write buffer="ROUT:OPEN:ALL", error in (no error)=w558) -> (VISA resource name out=w577:refnum<visa-resource-name>, error out=w576:errorcluster)  [unwired: 1 out]
            n130 = case shown="\"2400 and  2182\"" w595 {
              tunnel: w594 -> [_ w614 w619 _ _]
              tunnel: w593 -> [w610 w613 w620 _ _]
              tunnel: [w610 w612 w615 _ _] -> w561
              tunnel: w564 -> [_ _ w618 _ _]
              tunnel: w563 -> [w609 w611 w617 _ _]
              tunnel: [w609 w611 w616 _ _] -> w560
              frame "DAQ6510", Default {
              }
              frame "2400 Only" {
                n131 = call <instrlib>:"Close.vi"("error in (no error)"=w613, "VISA resource name"=w614) -> ("error out"=w612:errorcluster)  [unwired: 9 in]
              }
              frame "2400 and  2182" {
                n132 = call <instrlib>:"Close.vi"("error in (no error)"=w620, "VISA resource name"=w619) -> ("error out"=w615:errorcluster)  [unwired: 9 in]
                n133 = call <instrlib>:"Close.vi"("error in (no error)"=w617, "VISA resource name"=w618) -> ("error out"=w616:errorcluster)  [unwired: 9 in]
              }
              frame "SR830" {
              }
              frame "SR830 and 6221" {
              }
            }
            n134 = call <instrlib>:"Close.vi"("error in (no error)"=w576, "VISA resource name"=w577) -> ("error out"=w557:errorcluster)  [unwired: 9 in]
            n135 = call "save measurements.vi"("Save path"=w582, "Measurements In"=w562) -> ()  [unwired: 12 in, 2 out]
            n136 = Build Array(w557, w561, w560) -> (→"Comms Errors":errorcluster[])
          }
        }
        n137 = case shown="\"2400 Only\"" "Radio Buttons" {
          tunnel: [w541 FALSE w545 w546 w548] -> w534
          tunnel: [w541 w543 w545 w546 FALSE] -> w533
          tunnel: [TRUE w543 w545 TRUE w548] -> w529
          tunnel: [w541 w543 w545 w546 w548] -> w528
          frame "DAQ6510", Default {
            w541 = FALSE
          }
          frame "2400 Only" {
            w543 = TRUE
          }
          frame "2400 and  2182" {
            w545 = TRUE
          }
          frame "SR830" {
            w546 = FALSE
          }
          frame "SR830 and 6221" {
            w548 = TRUE
          }
        }
        n138 = property on="Measurement Repeats" class="DigNum (strict)"("Visible"=w529) -> ()  [unwired: 2 in, 2 out]
        n139 = property on="Current (µA)" class="DigNum (strict)"("Visible"=w533) -> ()  [unwired: 2 in, 2 out]
        n140 = property on="Measure Instrument" class="VISAName"("Visible"=w534) -> ()  [unwired: 2 in, 2 out]
        n141 = property on="Compliance voltage (V)" class="DigNum (strict)"("Visible"=w528) -> ()  [unwired: 2 in, 2 out]
      }
      frame 3 {
        # "Magnetic Op."
      }
      frame 4 {
        # "Calculations"
        # "Save File - saves collected data into a (csv) file and asks for a file path if not already given"
        n142 = Look In Map(map=w844, key="Resistance") -> (value=w842:dbl[])  [unwired: 1 in, 1 out]
        n143 = Build Array("Top Film R est.", "Bottm Film R est.", "RA est.") -> (w852:dbl[])
        n144 = case shown="True" "Fit Data" {
          tunnel: w847 -> [_ w872]
          tunnel: w852 -> [_ w870]
          tunnel: [dbl[] [0.0, 0.0, 0.0] w861] -> w849
          tunnel: w842 -> [_ w859]
          frame False {
          }
          frame True {
            # "Calculated R"
            # "Mean probe spacing"
            n145 = Index Array(array=w872, index (col)=4 ("disabled index (col)")) -> (element=w871:i64[])  [unwired: 1 in]
            n146 = vi-ref "modelFunction.vi"() -> (w869:refnum<vi>)
            n147 = call-poly <vilib>:"Nonlinear Curve Fit.vi"("Y"=w859, "f(x,a)"=w869, "X"=w871, "initial parameters"=w870) -> ("best fit parameters"=w861:dbl[], "error out"=→"error out (fitting model)":errorcluster)  [unwired: 6 in, 4 out]
            n148 = Index Array(array=w861, index=0) -> (element=→"Top Film R":dbl)
            n149 = Index Array(array=w861, index=1) -> (element=→"Bottom Film R":dbl)
            n150 = Index Array(array=w861, index=2) -> (element=→"RA":dbl)
          }
        }
        n151 = case shown="True" "Save Filr" {
          tunnel: w847 -> [_ w893]
          tunnel: string[] ["I+", "V+", "V-", "I-", "x (mean probe spacing)", "V", "I (µA)", "R (=V/I)"] -> [_ w889]
          tunnel: string[] ["R (t)", "R (b)", "RA"] -> [_ w881]
          tunnel: w849 -> [_ w874]
          tunnel: w845 -> [_ w873]
          frame False {
          }
          frame True {
            n152 = call-poly <vilib>:"Write Delimited Spreadsheet.vi"("file path (dialog if empty)"=w873, "1D data"=w889, "delimiter (\\t)"="," ("delimiter (\\t)")) -> ("new file path (Not A Path if cancelled)"=w891:path, "error out"=w890:errorcluster)  [unwired: 11 in]
            n153 = call-poly <vilib>:"Write Delimited Spreadsheet.vi"("file path (dialog if empty)"=w891, "format (%d)"="%.6f" ("format (%.3f)"), "2D data"=w893, "append to file? (new file:F)"=TRUE, "error in (no error)"=w890, "delimiter (\\t)"="," ("delimiter (\\t)")) -> ("new file path (Not A Path if cancelled)"=w883:path, "error out"=w882:errorcluster)  [unwired: 8 in]
            n154 = call-poly <vilib>:"Write Delimited Spreadsheet.vi"("file path (dialog if empty)"=w883, "format (%s)"="%.6f" ("format (%.3f)"), "1D data"=w881, "append to file? (new file:F)"=TRUE, "error in (no error)"=w882, "delimiter (\\t)"="," ("delimiter (\\t)")) -> ("new file path (Not A Path if cancelled)"=w876:path, "error out"=w875:errorcluster)  [unwired: 8 in]
            n155 = call-poly <vilib>:"Write Delimited Spreadsheet.vi"("file path (dialog if empty)"=w876, "format (%.3f)"="%.6f", "1D data"=w874, "append to file? (new file:F)"=TRUE, "error in (no error)"=w875, "delimiter (\\t)"="," ("delimiter (\\t)")) -> ("error out"=→"error file out":errorcluster)  [unwired: 8 in, 1 out]
          }
        }
        "Measurements Map Out" <- w844
      }
    }
    n156 = case shown="False" "Exit Camera 2" {
      tunnel: ["" "Exit camera"] -> w135
      frame False {
      }
      frame True {
      }
    }
    n157 = case shown="False" "Init Camera 2" {
      tunnel: ["" "Init camera"] -> w138
      frame False {
      }
      frame True {
      }
    }
    n158 = case shown="False" "Init Camera" {
      tunnel: ["" "Init camera"] -> w151
      frame False {
      }
      frame True {
      }
    }
    n159 = case shown="False" "Exit Camera" {
      tunnel: ["" "Exit camera"] -> w148
      frame False {
      }
      frame True {
      }
    }
    n160 = property on="Image first camera" class="Pict"("ZoomFactor"=0.175) -> ()  [unwired: 2 in, 2 out]
    n161 = property on="Image second camera" class="Pict"("ZoomFactor"=0.175) -> ()  [unwired: 2 in, 2 out]
    n162 = Concatenate Strings(w138, w135) -> (w137:string)
    n163 = Concatenate Strings(w151, w148) -> (w150:string)
    n164 = case shown="\"Init camera\"" w137 {
      tunnel: w128 -> [w279 w310 w375]
      tunnel: w127 -> [w280 w309 w374]
      tunnel: [w289 w312 w353] -> w130
      tunnel: [w290 w311 w354] -> w134
      tunnel: [TRUE FALSE FALSE] -> w132
      frame "Exit camera" {
        # "Close .Net Referenz"
        # "Is acquisition running?"
        # "Stop Acquisition"
        # "Close Camera"
        n165 = control-ref of="Init Camera 2"() -> (w274:refnum<vi>)
        n166 = control-ref of="Exit Camera 2"() -> (w273:refnum<vi>)
        n167 = property class="Camera"(reference=w279, error in=w280) -> (error out=w288:errorcluster, "Acquisition"=w287:refnum<k24>)  [unwired: 1 out]
        n168 = property class="Bool"(reference=w274, "Disabled"=u8 0 ("Deaktiviert")) -> ()  [unwired: 1 in, 2 out]
        n169 = property class="Bool"(reference=w273, "Disabled"=u8 2 ("Deaktiviert")) -> ()  [unwired: 1 in, 2 out]
        n170 = invoke class="Acquisition" method="HasStarted"(reference=w287, error in=w288) -> (reference out=w281:refnum<k24>, error out=w284:errorcluster, "bValue"=w286:bool)  [unwired: 2 in, 1 out]
        n171 = invoke class="Acquisition" method="ToString"(reference=w281, error in=w284) -> (error out=w283:errorcluster, "ToString"=w282:string)  [unwired: 1 in, 1 out]
        n172 = call <instrlib>:"Error_Handling.vi"("Error String"=w282, "Error In"=w283) -> ("Error Out"=w285:errorcluster)  [unwired: 9 in]
        n173 = case shown="True" w286 {
          tunnel: [w298 w307] -> w277
          tunnel: w285 -> [w298 w308]
          tunnel: w279 -> [w297 w299]
          tunnel: [w297 w299] -> w278
          frame False {
          }
          frame True {
            n174 = property class="Camera"(reference=w299, error in=w308) -> (error out=w303:errorcluster, "Acquisition"=w304:refnum<k24>)  [unwired: 1 out]
            n175 = invoke class="Acquisition" method="Stop"(reference=w304, error in=w303) -> (reference out=w301:refnum<k24>, error out=w302:errorcluster, "Stop"=w300:i32)  [unwired: 1 in]
            n176 = invoke class="Acquisition" method="ToString"(reference=w301, error in=w302) -> (error out=w306:errorcluster, "ToString"=w305:string)  [unwired: 1 in, 1 out]
            n177 = call <instrlib>:"Error_Handling.vi"("Error Code"=w300, "Error String"=w305, "Error In"=w306) -> ("Error Out"=w307:errorcluster)  [unwired: 8 in]
          }
        }
        n178 = invoke class="Camera" method="Exit"(reference=w278, error in=w277) -> (reference out=w289:refnum<k24>, error out=w293:errorcluster, "Exit"=w292:i32)  [unwired: 1 in]
        n179 = invoke class="Camera" method="ToString"(reference=w289, error in=w293) -> (error out=w294:errorcluster, "ToString"=w295:string)  [unwired: 1 in, 1 out]
        n180 = call <instrlib>:"Error_Handling.vi"("Error Code"=w292, "Error String"=w295, "Error In"=w294) -> ("Error Out"=w291:errorcluster)  [unwired: 8 in]
        n181 = Close Reference ("Close Referenz")(reference=w289, error in (no error)=w291) -> (error out=w290:errorcluster)
      }
      frame Default {
        # "Has acquisition started?"
        # "Show Image"
        n182 = property class="Camera"(reference=w310, error in=w309) -> (error out=w321:errorcluster, "Acquisition"=w320:refnum<k24>)  [unwired: 1 out]
        n183 = invoke class="Acquisition" method="HasStarted"(reference=w320, error in=w321) -> (reference out=w316:refnum<k24>, error out=w315:errorcluster, "HasStarted"=w314:i32, "bValue"=w319:bool)  [unwired: 2 in]
        n184 = invoke class="Acquisition" method="ToString"(reference=w316, error in=w315) -> (error out=w318:errorcluster, "ToString"=w317:string)  [unwired: 1 in, 1 out]
        n185 = call <instrlib>:"Error_Handling.vi"("Error Code"=w314, "Error String"=w317, "Error In"=w318) -> ("Error Out"=w313:errorcluster)  [unwired: 8 in]
        n186 = case shown="False" w319 {
          tunnel: [w324 w330] -> w311
          tunnel: w313 -> [w324 w329]
          tunnel: w310 -> [w323 w325]
          tunnel: [w323 w325] -> w312
          frame False {
          }
          frame True {
            # "Memory"
            n187 = property class="Camera"(reference=w325, error in=w329) -> (error out=w332:errorcluster, "Memory"=w333:refnum<k24>)  [unwired: 1 out]
            n188 = invoke class="Memory" method="GetActive"(reference=w333, error in=w332) -> (reference out=w339:refnum<k24>, error out=w338:errorcluster, "GetActive"=w340:i32, "s32MemId"=w331:i32)  [unwired: 2 in]
            n189 = invoke class="Memory" method="ToString"(reference=w339, error in=w338) -> (error out=w336:errorcluster, "ToString"=w337:string)  [unwired: 1 in, 1 out]
            n190 = call <instrlib>:"Error_Handling.vi"("Error Code"=w340, "Error String"=w337, "Error In"=w336) -> ("Error Out"=w341:errorcluster)  [unwired: 8 in]
            n191 = property class="Camera"(reference=w325, error in=w341) -> (error out=w335:errorcluster, "Memory"=w334:refnum<k24>)  [unwired: 1 out]
            n192 = invoke class="Memory" method="CopyToArray"(reference=w334, error in=w335, "s32MemId"=w331) -> (reference out=w344:refnum<k24>, error out=w345:errorcluster, "CopyToArray"=w346:i32, "u8Image"=w326:u8[])  [unwired: 2 in, 1 out]
            n193 = invoke class="Memory" method="ToString"(reference=w344, error in=w345) -> (error out=w342:errorcluster, "ToString"=w343:string)  [unwired: 1 in, 1 out]
            n194 = call <instrlib>:"Error_Handling.vi"("Error Code"=w346, "Error String"=w343, "Error In"=w342) -> ("Error Out"=w327:errorcluster)  [unwired: 8 in]
            n195 = call <instrlib>:"ArrayToImage.vi"("Error In"=w327, "InArray"=w326, ".NET (Reference)"=w325) -> ("Error Out"=w330:errorcluster, "Image"=→"Image second camera":picture)  [unwired: 7 in]
          }
        }
      }
      frame "Init camera" {
        w355 = 1 items=["IS_DONT_WAIT", "IS_WAIT"] ("Wait")
        w382 = 0 items=["RGB 32"=0, "RGB 24"=1, "Y8 Monochrom"=6] ("Mode")
        # "SubVI Example for \nGetDefault Timing"
        # "SubVI Example for \nMemory allocation"
        # "SubVI Example for \nTiming"
        # "SubVI Example for \nCamera Init"
        # "Pixelformat"
        n196 = control-ref of="Init Camera 2"() -> (w350:refnum<vi>)
        n197 = control-ref of="Exit Camera 2"() -> (w348:refnum<vi>)
        n198 = property class="Bool"(reference=w350, "Disabled"=u8 2 ("Deaktiviert")) -> ()  [unwired: 1 in, 2 out]
        n199 = property class="Bool"(reference=w348, "Disabled"=u8 0 ("Deaktiviert")) -> ()  [unwired: 1 in, 2 out]
        n200 = call <instrlib>:"SubVI_Example_CameraInit.vi"("Error In"=w374, "Camera ID"="Camera ID 3", "Init Camera Flag"=TRUE, ".NET (Reference)"=w375) -> ("Error Out"=w379:errorcluster, ".NET (Reference)"=w353:refnum<k24>)  [unwired: 6 in]
        n201 = property class="Camera"(reference=w353, error in=w379) -> (error out=w380:errorcluster, "PixelFormat"=w381:refnum<k24>)  [unwired: 1 out]
        n202 = invoke class="PixelFormat" method="Set"(reference=w381, error in=w380, "mode"=w382) -> (reference out=w377:refnum<k24>, error out=w371:errorcluster, "Set"=w376:i32)  [unwired: 1 in, 1 out]
        n203 = invoke class="PixelFormat" method="ToString"(reference=w377, error in=w371) -> (error out=w370:errorcluster, "ToString"=w378:string)  [unwired: 1 in, 1 out]
        n204 = call <instrlib>:"Error_Handling.vi"("Error Code"=w376, "Error String"=w378, "Error In"=w370) -> ("Error Out"=w367:errorcluster)  [unwired: 8 in]
        n205 = call <instrlib>:"SubVI_Example_GetDefault_Timing.vi"(".NET (Reference)"=w353, "Error In"=w367) -> ("Pixelclock"=w364:i32, "Exposure time"=w365:dbl, "Framerate"=w366:dbl, "Error Out"=w363:errorcluster)  [unwired: 10 in]
        n206 = call <instrlib>:"SubVI_Example_Timing.vi"(".NET (Reference)"=w353, "Pixelclock"=w364, "Exposure time"=w365, "Framerate"=w366, "Error In"=w363) -> ("Error Out"=w369:errorcluster)  [unwired: 7 in, 3 out]
        n207 = call <instrlib>:"SubVI_Example_MemoryAllocation.vi"(".NET (Reference)"=w353, "Error In"=w369) -> ("Serial Number"=→"Serial Number 2":string, "Error Out"=w352:errorcluster)  [unwired: 13 in, 3 out]
        n208 = property class="Camera"(reference=w353, error in=w352) -> (error out=w361:errorcluster, "Acquisition"=w362:refnum<k24>)  [unwired: 1 out]
        n209 = invoke class="Acquisition" method="Capture"(reference=w362, error in=w361, "param"=w355) -> (reference out=w357:refnum<k24>, error out=w358:errorcluster, "Capture"=w356:i32)  [unwired: 1 in, 1 out]
        n210 = invoke class="Acquisition" method="ToString"(reference=w357, error in=w358) -> (error out=w360:errorcluster, "ToString"=w359:string)  [unwired: 1 in, 1 out]
        n211 = call <instrlib>:"Error_Handling.vi"("Error Code"=w356, "Error String"=w359, "Error In"=w360) -> ("Error Out"=w354:errorcluster)  [unwired: 8 in]
      }
    }
    n212 = case shown="Default" w150 {
      tunnel: w141 -> [w393 w424 w489]
      tunnel: w140 -> [w394 w423 w488]
      tunnel: [w403 w426 w468] -> w143
      tunnel: [w404 w425 w469] -> w147
      tunnel: [TRUE FALSE FALSE] -> w145
      frame "Exit camera" {
        # "Close .Net Referenz"
        # "Is acquisition running?"
        # "Stop Acquisition"
        # "Close Camera"
        n213 = control-ref of="Init Camera"() -> (w388:refnum<vi>)
        n214 = control-ref of="Exit Camera"() -> (w387:refnum<vi>)
        n215 = property class="Camera"(reference=w393, error in=w394) -> (error out=w402:errorcluster, "Acquisition"=w401:refnum<k24>)  [unwired: 1 out]
        n216 = property class="Bool"(reference=w388, "Disabled"=u8 0 ("Deaktiviert")) -> ()  [unwired: 1 in, 2 out]
        n217 = property class="Bool"(reference=w387, "Disabled"=u8 2 ("Deaktiviert")) -> ()  [unwired: 1 in, 2 out]
        n218 = invoke class="Acquisition" method="HasStarted"(reference=w401, error in=w402) -> (reference out=w395:refnum<k24>, error out=w398:errorcluster, "bValue"=w400:bool)  [unwired: 2 in, 1 out]
        n219 = invoke class="Acquisition" method="ToString"(reference=w395, error in=w398) -> (error out=w397:errorcluster, "ToString"=w396:string)  [unwired: 1 in, 1 out]
        n220 = call <instrlib>:"Error_Handling.vi"("Error String"=w396, "Error In"=w397) -> ("Error Out"=w399:errorcluster)  [unwired: 9 in]
        n221 = case shown="True" w400 {
          tunnel: [w412 w421] -> w391
          tunnel: w399 -> [w412 w422]
          tunnel: w393 -> [w411 w413]
          tunnel: [w411 w413] -> w392
          frame False {
          }
          frame True {
            n222 = property class="Camera"(reference=w413, error in=w422) -> (error out=w417:errorcluster, "Acquisition"=w418:refnum<k24>)  [unwired: 1 out]
            n223 = invoke class="Acquisition" method="Stop"(reference=w418, error in=w417) -> (reference out=w415:refnum<k24>, error out=w416:errorcluster, "Stop"=w414:i32)  [unwired: 1 in]
            n224 = invoke class="Acquisition" method="ToString"(reference=w415, error in=w416) -> (error out=w420:errorcluster, "ToString"=w419:string)  [unwired: 1 in, 1 out]
            n225 = call <instrlib>:"Error_Handling.vi"("Error Code"=w414, "Error String"=w419, "Error In"=w420) -> ("Error Out"=w421:errorcluster)  [unwired: 8 in]
          }
        }
        n226 = invoke class="Camera" method="Exit"(reference=w392, error in=w391) -> (reference out=w403:refnum<k24>, error out=w407:errorcluster, "Exit"=w406:i32)  [unwired: 1 in]
        n227 = invoke class="Camera" method="ToString"(reference=w403, error in=w407) -> (error out=w408:errorcluster, "ToString"=w409:string)  [unwired: 1 in, 1 out]
        n228 = call <instrlib>:"Error_Handling.vi"("Error Code"=w406, "Error String"=w409, "Error In"=w408) -> ("Error Out"=w405:errorcluster)  [unwired: 8 in]
        n229 = Close Reference ("Close Referenz")(reference=w403, error in (no error)=w405) -> (error out=w404:errorcluster)
      }
      frame Default {
        # "Has acquisition started?"
        n230 = property class="Camera"(reference=w424, error in=w423) -> (error out=w435:errorcluster, "Acquisition"=w434:refnum<k24>)  [unwired: 1 out]
        n231 = invoke class="Acquisition" method="HasStarted"(reference=w434, error in=w435) -> (reference out=w430:refnum<k24>, error out=w429:errorcluster, "HasStarted"=w428:i32, "bValue"=w433:bool)  [unwired: 2 in]
        n232 = invoke class="Acquisition" method="ToString"(reference=w430, error in=w429) -> (error out=w432:errorcluster, "ToString"=w431:string)  [unwired: 1 in, 1 out]
        n233 = call <instrlib>:"Error_Handling.vi"("Error Code"=w428, "Error String"=w431, "Error In"=w432) -> ("Error Out"=w427:errorcluster)  [unwired: 8 in]
        n234 = case shown="True" w433 {
          tunnel: [w438 w444] -> w425
          tunnel: w427 -> [w438 w443]
          tunnel: w424 -> [w437 w441]
          tunnel: [w437 w441] -> w426
          frame False {
            # "Show Image"
          }
          frame True {
            # "Memory"
            n235 = property class="Camera"(reference=w441, error in=w443) -> (error out=w446:errorcluster, "Memory"=w447:refnum<k24>)  [unwired: 1 out]
            n236 = invoke class="Memory" method="GetActive"(reference=w447, error in=w446) -> (reference out=w453:refnum<k24>, error out=w452:errorcluster, "GetActive"=w454:i32, "s32MemId"=w445:i32)  [unwired: 2 in]
            n237 = invoke class="Memory" method="ToString"(reference=w453, error in=w452) -> (error out=w450:errorcluster, "ToString"=w451:string)  [unwired: 1 in, 1 out]
            n238 = call <instrlib>:"Error_Handling.vi"("Error Code"=w454, "Error String"=w451, "Error In"=w450) -> ("Error Out"=w455:errorcluster)  [unwired: 8 in]
            n239 = property class="Camera"(reference=w441, error in=w455) -> (error out=w449:errorcluster, "Memory"=w448:refnum<k24>)  [unwired: 1 out]
            n240 = invoke class="Memory" method="CopyToArray"(reference=w448, error in=w449, "s32MemId"=w445) -> (reference out=w458:refnum<k24>, error out=w459:errorcluster, "CopyToArray"=w460:i32, "u8Image"=w440:u8[])  [unwired: 2 in, 1 out]
            n241 = invoke class="Memory" method="ToString"(reference=w458, error in=w459) -> (error out=w456:errorcluster, "ToString"=w457:string)  [unwired: 1 in, 1 out]
            n242 = call <instrlib>:"Error_Handling.vi"("Error Code"=w460, "Error String"=w457, "Error In"=w456) -> ("Error Out"=w442:errorcluster)  [unwired: 8 in]
            n243 = call <instrlib>:"ArrayToImage.vi"("Error In"=w442, "InArray"=w440, ".NET (Reference)"=w441) -> ("Error Out"=w444:errorcluster, "Image"=→"Image first camera":picture)  [unwired: 7 in]
          }
        }
      }
      frame "Init camera" {
        w470 = 1 items=["IS_DONT_WAIT", "IS_WAIT"] ("Wait")
        w496 = 0 items=["RGB 32"=0, "RGB 24"=1, "Y8 Monochrom"=6] ("Mode")
        # "SubVI Example for \nGetDefault Timing"
        # "SubVI Example for \nMemory allocation"
        # "SubVI Example for \nTiming"
        # "SubVI Example for \nCamera Init"
        # "Pixelformat"
        n244 = control-ref of="Init Camera"() -> (w464:refnum<vi>)
        n245 = control-ref of="Exit Camera"() -> (w462:refnum<vi>)
        n246 = call <instrlib>:"SubVI_Example_CameraInit.vi"("Error In"=w488, "Camera ID"="Camera ID 1", "Init Camera Flag"=TRUE, ".NET (Reference)"=w489) -> ("Error Out"=w493:errorcluster, ".NET (Reference)"=w468:refnum<k24>)  [unwired: 6 in]
        n247 = property class="Bool"(reference=w464, "Disabled"=u8 2 ("Deaktiviert")) -> ()  [unwired: 1 in, 2 out]
        n248 = property class="Bool"(reference=w462, "Disabled"=u8 0 ("Deaktiviert")) -> ()  [unwired: 1 in, 2 out]
        n249 = property class="Camera"(reference=w468, error in=w493) -> (error out=w494:errorcluster, "PixelFormat"=w495:refnum<k24>)  [unwired: 1 out]
        n250 = invoke class="PixelFormat" method="Set"(reference=w495, error in=w494, "mode"=w496) -> (reference out=w491:refnum<k24>, error out=w485:errorcluster, "Set"=w490:i32)  [unwired: 1 in, 1 out]
        n251 = invoke class="PixelFormat" method="ToString"(reference=w491, error in=w485) -> (error out=w484:errorcluster, "ToString"=w492:string)  [unwired: 1 in, 1 out]
        n252 = call <instrlib>:"Error_Handling.vi"("Error Code"=w490, "Error String"=w492, "Error In"=w484) -> ("Error Out"=w481:errorcluster)  [unwired: 8 in]
        n253 = call <instrlib>:"SubVI_Example_GetDefault_Timing.vi"(".NET (Reference)"=w468, "Error In"=w481) -> ("Pixelclock"=w478:i32, "Exposure time"=w479:dbl, "Framerate"=w480:dbl, "Error Out"=w466:errorcluster)  [unwired: 10 in]
        n254 = call <instrlib>:"SubVI_Example_Timing.vi"(".NET (Reference)"=w468, "Pixelclock"=w478, "Exposure time"=w479, "Framerate"=w480, "Error In"=w466) -> ("Error Out"=w483:errorcluster)  [unwired: 7 in, 3 out]
        n255 = call <instrlib>:"SubVI_Example_MemoryAllocation.vi"(".NET (Reference)"=w468, "Error In"=w483) -> ("Serial Number"=→"Serial Number 1":string, "Error Out"=w467:errorcluster)  [unwired: 13 in, 3 out]
        n256 = property class="Camera"(reference=w468, error in=w467) -> (error out=w476:errorcluster, "Acquisition"=w477:refnum<k24>)  [unwired: 1 out]
        n257 = invoke class="Acquisition" method="Capture"(reference=w477, error in=w476, "param"=w470) -> (reference out=w472:refnum<k24>, error out=w473:errorcluster, "Capture"=w471:i32)  [unwired: 1 in, 1 out]
        n258 = invoke class="Acquisition" method="ToString"(reference=w472, error in=w473) -> (error out=w475:errorcluster, "ToString"=w474:string)  [unwired: 1 in, 1 out]
        n259 = call <instrlib>:"Error_Handling.vi"("Error Code"=w471, "Error String"=w474, "Error In"=w475) -> ("Error Out"=w469:errorcluster)  [unwired: 8 in]
      }
    }
    n260 = case shown="False" "steps /\n continuous \ntoggle" {
      tunnel: w114 -> [w171 w247]
      tunnel: w113 -> [w170 w246]
      tunnel: [w189 w253] -> w112
      tunnel: [w162 w259] -> w102
      tunnel: "up a1" -> [w188 w255]
      tunnel: "down a1" -> [w186 w254]
      tunnel: "up all" -> [w169 w242]
      tunnel: "down all" -> [w168 w243]
      tunnel: "down a3" -> [w176 w251]
      tunnel: "up a3" -> [w177 w250]
      tunnel: "down a2" -> [w174 w245]
      tunnel: "up a2" -> [w175 w244]
      tunnel: w107 -> [_ w257]
      tunnel: [_ w258] -> w111
      tunnel: [_ w238] -> w110
      tunnel: w106 -> [_ w235]
      tunnel: [_ w236] -> w108
      tunnel: w104 -> [_ w233]
      tunnel: [_ w237] -> w109
      tunnel: w105 -> [_ w234]
      frame False {
        n261 = flat-sequence {
          tunnel: w171 -> [w204]
          tunnel: w170 -> [w207]
          tunnel: w177 -> [w202]
          tunnel: "a3" ("Combo Box") -> [w200]
          tunnel: "Step size" -> [w203]
          tunnel: w176 -> [w201]
          tunnel: [w206] -> w180
          tunnel: [w205] -> w179
          tunnel: [w209] -> _
          tunnel: [w210] -> w164
          tunnel: w180 -> [w210]
          tunnel: w179 -> [w209]
          frame #0 {
            n262 = call "Picomotor step single.vi"("Step size"=w203, "Combo Box"=w200, "error in (no error)"=w207, "down a1"=w201, "up a1"=w202, "VISA Refnum in"=w204) -> ("error out"=w206:errorcluster, "VISA Refnum out"=w205:refnum<visa-resource-name>)  [unwired: 4 in]
          }
          frame #1 {
            n263 = Wait (ms)(milliseconds to wait=u32 100) -> ()  [unwired: 1 out]
          }
        }
        n264 = flat-sequence {
          tunnel: w171 -> [w226]
          tunnel: w170 -> [w229]
          tunnel: w188 -> [w224]
          tunnel: "a1" ("Combo Box") -> [w222]
          tunnel: "Step size" -> [w225]
          tunnel: w186 -> [w223]
          tunnel: [w228] -> w185
          tunnel: [w227] -> w184
          tunnel: [w231] -> w189
          tunnel: [w232] -> w166
          tunnel: w185 -> [w232]
          tunnel: w184 -> [w231]
          frame #0 {
            n265 = call "Picomotor step single.vi"("Step size"=w225, "Combo Box"=w222, "error in (no error)"=w229, "down a1"=w223, "up a1"=w224, "VISA Refnum in"=w226) -> ("error out"=w228:errorcluster, "VISA Refnum out"=w227:refnum<visa-resource-name>)  [unwired: 4 in]
          }
          frame #1 {
            n266 = Wait (ms)(milliseconds to wait=u32 100) -> ()  [unwired: 1 out]
          }
        }
        n267 = flat-sequence {
          tunnel: w171 -> [w215]
          tunnel: w170 -> [w218]
          tunnel: w175 -> [w213]
          tunnel: "a2" ("Combo Box") -> [w211]
          tunnel: "Step size" -> [w214]
          tunnel: w174 -> [w212]
          tunnel: [w217] -> w183
          tunnel: [w216] -> w182
          tunnel: [w220] -> _
          tunnel: [w221] -> w165
          tunnel: w183 -> [w221]
          tunnel: w182 -> [w220]
          frame #0 {
            n268 = call "Picomotor step single.vi"("Step size"=w214, "Combo Box"=w211, "error in (no error)"=w218, "down a1"=w212, "up a1"=w213, "VISA Refnum in"=w215) -> ("error out"=w217:errorcluster, "VISA Refnum out"=w216:refnum<visa-resource-name>)  [unwired: 4 in]
          }
          frame #1 {
            n269 = Wait (ms)(milliseconds to wait=u32 100) -> ()  [unwired: 1 out]
          }
        }
        n270 = flat-sequence {
          tunnel: [w196] -> w173
          tunnel: [w195] -> w172
          tunnel: w171 -> [w194]
          tunnel: w170 -> [w193]
          tunnel: w169 -> [w192]
          tunnel: w168 -> [w191]
          tunnel: "Step size" -> [w190]
          tunnel: [w198] -> _
          tunnel: [w199] -> w163
          tunnel: w173 -> [w199]
          tunnel: w172 -> [w198]
          frame #0 {
            n271 = call "Picomotor step multi.vi"("Step size"=w190, "error in (no error)"=w193, "down a1"=w191, "up a1"=w192, "VISA Refnum in"=w194) -> ("error out"=w196:errorcluster, "VISA Refnum out"=w195:refnum<visa-resource-name>)  [unwired: 5 in]
          }
          frame #1 {
            n272 = Wait (ms)(milliseconds to wait=u32 100) -> ()  [unwired: 1 out]
          }
        }
        n273 = Merge Errors(w166, w165, w164, w163) -> (w162:errorcluster)
      }
      frame True {
        n274 = call "Picomotor single motor continuous.vi"("Enum"=w257, "Combo Box"="a1", "error in (no error)"=w246, "down"=w254, "up"=w255, "VISA Refnum in"=w247) -> ("error out"=w252:errorcluster, "Numeric"=w258:i32, "VISA Refnum out"=w253:refnum<visa-resource-name>)  [unwired: 3 in]
        n275 = call "Picomotor single motor continuous.vi"("Enum"=w234, "Combo Box"="a3", "error in (no error)"=w246, "down"=w251, "up"=w250, "VISA Refnum in"=w247) -> ("error out"=w240:errorcluster, "Numeric"=w237:i32)  [unwired: 3 in, 1 out]
        n276 = call "Picomotor single motor continuous.vi"("Enum"=w235, "Combo Box"="a2", "error in (no error)"=w246, "down"=w245, "up"=w244, "VISA Refnum in"=w247) -> ("error out"=w241:errorcluster, "Numeric"=w238:i32)  [unwired: 3 in, 1 out]
        n277 = call "Picomotor all motors continuous.vi"("Enum"=w233, "error in (no error)"=w246, "down"=w243, "up"=w242, "VISA Refnum in"=w247) -> ("error out"=w239:errorcluster, "Numeric"=w236:i32)  [unwired: 4 in, 1 out]
        n278 = Merge Errors(w252, w241, w240, w239) -> (w259:errorcluster)
      }
    }
    n279 = call <instrlib>:"SubVI_Example_SyncEventLoop.vi"("Error In"=w134, "use sync"=w132, ".NET (Reference)"=w130) -> ("Error Out"=w129:errorcluster, "Synchronize (ms)"=w133:dbl)  [unwired: 7 in]
    "Error Camera 2" <- w129
    n280 = call <instrlib>:"SubVI_Example_SyncEventLoop.vi"("Error In"=w147, "use sync"=w145, ".NET (Reference)"=w143) -> ("Error Out"=w142:errorcluster, "Synchronize (ms)"=w146:dbl)  [unwired: 7 in]
    "Error Camera 1" <- w142
    n281 = Wait Until Next ms Multiple(millisecond multiple=w146) -> ()  [unwired: 1 out]
    n282 = Wait Until Next ms Multiple(millisecond multiple=w133) -> ()  [unwired: 1 out]
    n283 = case shown="False" "stop" {
      tunnel: w112 -> [w262 w267]
      tunnel: w102 -> [w261 w266]
      tunnel: [w262 w265] -> w101
      tunnel: [w261 w264] -> w103
      tunnel: [w260 w263] -> w125
      tunnel: "stop" -> [w260 w263]
      frame False {
      }
      frame True {
        n284 = call "Picomotor Write.vi"("error in (no error)"=w266, "String 3"="sto", "VISA Refnum in"=w267) -> ("error out"=w264:errorcluster, "VISA Refnum out"=w265:refnum<visa-resource-name>)  [unwired: 6 in, 1 out]
      }
    }
    n285 = Merge Errors(w103, w102) -> (w126:errorcluster)
  }
  n286 = VISA Close(VISA resource name=w1, error in (no error)=w2) -> (error out=→"error":errorcluster)
